vi "Initialize Compiled Step.vi"(6 "Step Number":i32, 8 "error in (no error)":errorcluster, 10 "Step Values":T1, 11 "Output Sequencer in":refnum<class "Output Sequencer.lvclass">) -> (0 "error out":errorcluster, 2 "Compiled Step":T2, 3 "Output Sequencer out":refnum<class "Output Sequencer.lvclass">)   [LabVIEW 2024, in "Output Sequencer.lvlib" / "Output Sequencer.lvclass"]
uses:
  Output Sequencer.lvclass
  Types/Compiled Step.ctl
  <vilib>/LAVA/muParser/mupExpr/mupExpr.lvclass
  Types/Expression Data.ctl
  Settings UI/Types/Step Settings.ctl
  Settings UI/Settings UI.lvclass
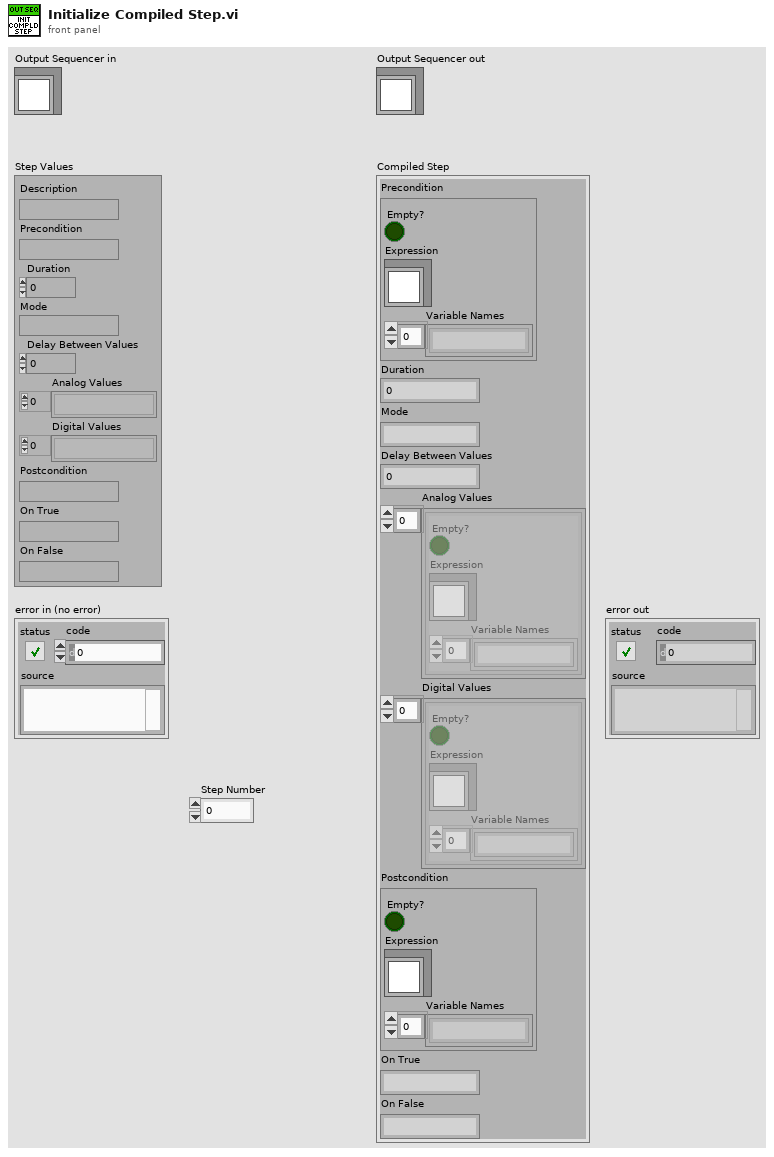
[diagram p1: front panel]
types:
  T1 = typedef "Output Sequencer.lvlib/Settings UI.lvclass/Step Settings.ctl" = cluster{"Description":string, "Precondition":string, "Duration":dbl, "Mode":string, "Delay Between Values":dbl, "Analog Values":string[], "Digital Values":string[], "Postcondition":string, "On True":string, "On False":string}
  T2 = typedef "Output Sequencer.lvlib/Output Sequencer.lvclass/Compiled Step.ctl" = cluster{"Precondition":T3, "Duration":dbl, "Mode":string, "Delay Between Values":dbl, "Analog Values":T3[], "Digital Values":T3[], "Postcondition":T3, "On True":string, "On False":string}
  T3 = typedef "Output Sequencer.lvlib/Output Sequencer.lvclass/Expression Data.ctl" = cluster{"Empty?":bool, "Expression":refnum<class "mupExpr.lvclass">, "Variable Names":string[]}
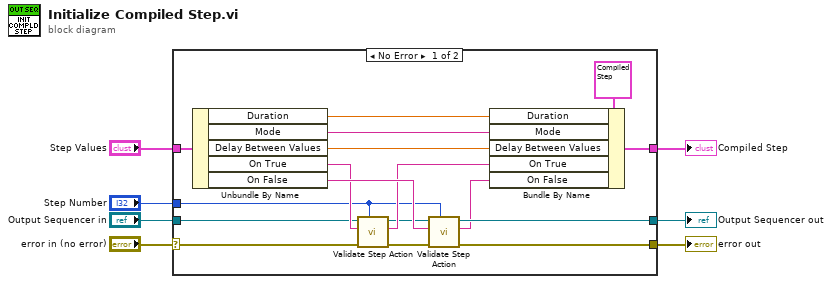
[diagram p0: block diagram]
diagram:
  n1 = case shown="No Error" "error in (no error)" {
    selector: "error in (no error)" -> [w9 w25]
    tunnel: [w24 _] -> w7
    tunnel: "Step Values" -> [w23 _]
    tunnel: "Output Sequencer in" -> [w10 w26]
    tunnel: [w17 w26] -> w4
    tunnel: [w18 w25] -> w2
    tunnel: "Step Number" -> [w8 _]
    frame No Error {
      n2 = Unbundle By Name(w23) -> ("Duration"=w21:dbl, "Mode"=w20:string, "Delay Between Values"=w19:dbl, "On True"=w14:string, "On False"=w16:string)
      n3 = call "Validate Step Action.vi"("Step Number"=w8, "error in (no error)"=w9, "Action in"=w14, "Output Sequencer in"=w10) -> ("error out"=w11:errorcluster, "Action out"=w13:string, "Output Sequencer out"=w12:refnum<class "Output Sequencer.lvclass">)  [unwired: 5 in]
      n4 = call "Validate Step Action.vi"("Step Number"=w8, "error in (no error)"=w11, "Action in"=w16, "Output Sequencer in"=w12) -> ("error out"=w18:errorcluster, "Action out"=w15:string, "Output Sequencer out"=w17:refnum<class "Output Sequencer.lvclass">)  [unwired: 5 in]
      n5 = Bundle By Name(cluster=T2 {"Precondition"={"Empty?"=FALSE, "Expression"=refnum, "Variable Names"=[]}, "Duration"=0.0, "Mode"="", "Delay Between Values"=0.0, "Analog Values"=[], "Digital Values"=[], "Postcondition"={"Empty?"=FALSE, "Expression"=refnum, "Variable Names"=[]}, "On True"="", "On False"=""} ("Compiled Step"), "Duration"=w21, "Mode"=w20, "Delay Between Values"=w19, "On True"=w13, "On False"=w15) -> (w24:T2)
    }
    frame Error {
    }
  }
  "Output Sequencer out" <- w4
  "Compiled Step" <- w7
  "error out" <- w2
